vi "ArmLiftControl2.vi"(11 "erronIn(d)":dbl) -> (2 "OnTarget":bool, 3 "motorOutput":dbl)   [LabVIEW 2020]
uses:
  <vilib>/Rock Robotics/WPI/ThirdParty/JAS_Junk/TrajLib/PIDController_AtSetpoint.vi
  <vilib>/Rock Robotics/WPI/ThirdParty/JAS_Junk/TrajLib/PIDController_SetPIDF.vi
  <vilib>/Rock Robotics/WPI/ThirdParty/JAS_Junk/TrajLib/PIDController_SetDerivativeFilter.vi
  <vilib>/Rock Robotics/WPI/ThirdParty/JAS_Junk/TrajLib/PIDController_SetIntegratorRange.vi
  <vilib>/Rock Robotics/WPI/ThirdParty/JAS_Junk/TrajLib/PIDController_SetTolerancePandV.vi
  <vilib>/Rock Robotics/WPI/ThirdParty/JAS_Junk/TrajLib/PIDController_DisableContinousInput.vi
  <vilib>/Rock Robotics/WPI/ThirdParty/JAS_Junk/TrajLib/PIDController_EnableContinousInput.vi
  <vilib>/Rock Robotics/WPI/ThirdParty/JAS_Junk/TrajLib/PIDController_Reset.vi
  <vilib>/Rock Robotics/WPI/ThirdParty/JAS_Junk/TrajLib/PIDController_New.vi
  <vilib>/Rock Robotics/WPI/ThirdParty/JAS_Junk/TrajLib/PIDController_SetOutputLimits.vi
  <vilib>/Rock Robotics/WPI/ThirdParty/JAS_Junk/TrajLib/PIDController_NewPeriod.vi
  <vilib>/Rock Robotics/SystemInterfaces/NetworkCommunication/NetComm_UsageReport_report.vi
  <vilib>/Rock Robotics/WPI/ThirdParty/JAS_Junk/TrajLib/Globals/Util_LibraryGlobals.vi
  <vilib>/Rock Robotics/WPI/ThirdParty/JAS_Junk/TrajLib/PIDController_AdvCalculate_FF_Sp_Pv.vi
  <vilib>/Rock Robotics/WPI/ThirdParty/JAS_Junk/TrajLib/Trajectory_Library.lvlib
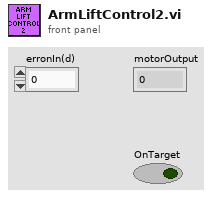
[diagram p1: front panel]
types:
  T1 = typedef "Trajectory_Library.lvlib/PID_ADV_LIMITS.ctl" = cluster{"MaxInput":dbl, "MinInput":dbl, "Continuous":bool, "MaxOutput":dbl, "MinOutput":dbl}
  T2 = typedef "Trajectory_Library.lvlib/PID_ADV_TUNING.ctl" = cluster{"Kf":dbl, "Kp":dbl, "Ki":dbl, "Kd":dbl, "MaximumIntegral":dbl, "MinimumIntegral":dbl, "Filter Derivative":bool}
  T3 = typedef "Trajectory_Library.lvlib/PID_ERROR_TOLERANCE.ctl" = cluster{"PositionTolerance":dbl, "VelocityTolerance":dbl}
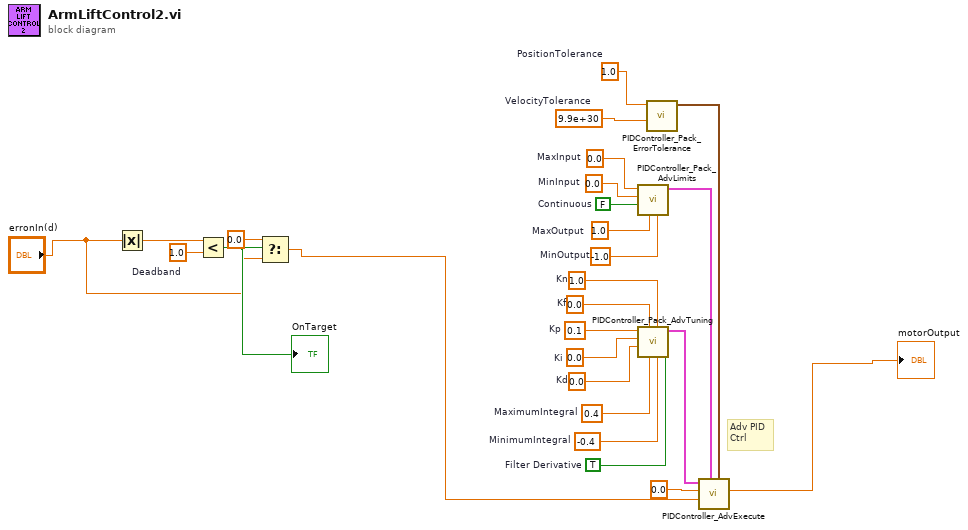
[diagram p0: block diagram]
diagram:
  w5 = 1.0  # Deadband
  w7 = 1.0  # PositionTolerance
  w8 = 9.9e+30  # VelocityTolerance
  w26 = 1.0  # Kn
  w25 = 0.1  # Kp
  w24 = 0.0  # Ki
  w23 = 0.0  # Kd
  w22 = 0.0  # Kf
  w21 = 0.4  # MaximumIntegral
  w20 = -0.4  # MinimumIntegral
  w19 = TRUE  # Filter Derivative
  w17 = 0.0  # MinInput
  w16 = FALSE  # Continuous
  w15 = 1.0  # MaxOutput
  w18 = -1.0  # MinOutput
  w14 = 0.0  # MaxInput
  # "Adv PID\nCtrl"
  n1 = Absolute Value(x="erronIn(d)") -> (abs(x)=w6:dbl)
  n2 = Less?(x=w6, y=w5) -> (x < y?=w3:bool)
  "OnTarget" <- w3
  n3 = Select(t=0.0, s=w3, f="erronIn(d)") -> (s? t:f=w4:dbl)
  n4 = call <vilib>:"PIDController_Pack_AdvLimits.vi"("MinOutput"=w18, "MaxOutput"=w15, "Continuous"=w16, "MinInput"=w17, "MaxInput"=w14) -> ("Adv PID Limits"=w12:T1)  [unwired: 6 in]
  n5 = call <vilib>:"PIDController_Pack_AdvTuning.vi"("Filter Derivative"=w19, "MinimumIntegral"=w20, "Kn"=w26, "MaximumIntegral"=w21, "Kf"=w22, "Kd"=w23, "Ki"=w24, "Kp"=w25) -> ("Adv PID Tuning"=w13:T2)  [unwired: 3 in]
  n6 = call <vilib>:"PIDController_Pack_ErrorTolerance.vi"("VelocityTolerance"=w8, "PositionTolerance"=w7) -> ("PID Error Tolerance"=w9:T3)  [unwired: 9 in]
  n7 = call <vilib>:"PIDController_AdvExecute.vi"("PID Error Tolerance"=w9, "Adv PID Limits"=w12, "SP-SetPoint"=w4, "PV-Measurement"=0.0, "Adv PID Tuning"=w13) -> ("CO-ControlOutput"=→"motorOutput":dbl)  [unwired: 4 in, 2 out]
